vi "requestStop.vi"(8 "error in (no error)":errorcluster, 11 "MsgUserEventStopMechanism In":refnum<class "MsgUETaskChannel.lvclass">) -> (0 "error out":errorcluster, 3 "MsgUserEventStopMechanism Out":refnum<class "MsgUETaskChannel.lvclass">)   [LabVIEW 2023, in "TLC_Daemon.lvlib" / "MsgUETaskChannel.lvclass"]
doc: "Triggers a stop request for a target task."
uses:
  MsgUETaskChannel.lvclass
  MsgUETaskChannel.lvclass/MsgUETaskChannel.ctl
  Ctrls/msg.ctl
  TLC_Daemon.lvlib
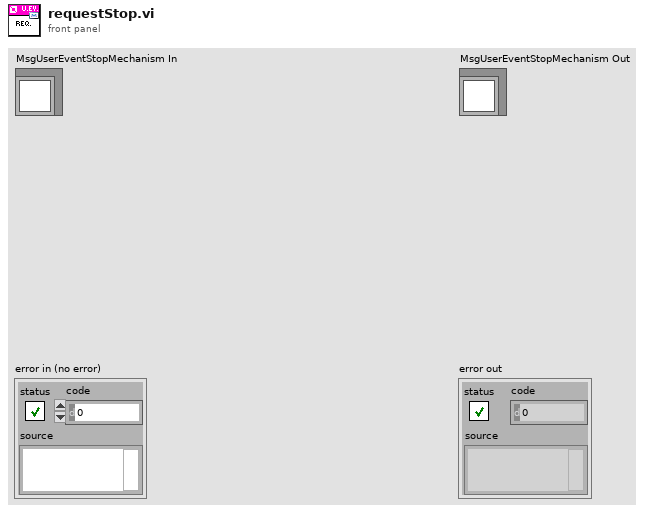
[diagram p1: front panel]
types:
  T1 = typedef "TLC_Daemon.lvlib/msg.ctl" = cluster{"message":string, "data":variant}
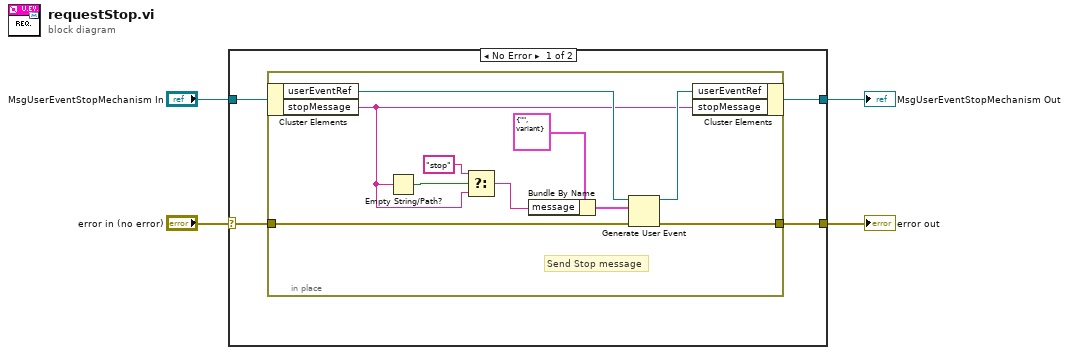
[diagram p0: block diagram]
diagram:
  n1 = case shown="No Error" "error in (no error)" {
    selector: "error in (no error)" -> [w7 w20]
    tunnel: [w6 w20] -> w3
    tunnel: "MsgUserEventStopMechanism In" -> [w8 w19]
    tunnel: [w5 w19] -> w1
    frame No Error {
      n2 = in-place {
        in-place-border: w7 -> [w16]
        in-place-border: [w15] -> w6
        # "Send Stop message"
        n3 = in-place-cluster #1(w8) -> ("userEventRef"=w18:refnum<user-event>, "stopMessage"=w11:string)
        n4 = Empty String/Path?(string/path=w11) -> (empty?=w12:bool)
        n5 = Select(t="stop", s=w12, f=w11) -> (s? t:f=w10:string)
        n6 = Bundle By Name(cluster=T1 {"message"="", "data"=variant} ("msg"), "message"=w10) -> (w14:T1)
        n7 = Generate User Event(user event=w18, event data cluster=w14, error in=w16) -> (user event out=w17:refnum<user-event>, error out=w15:errorcluster)  [unwired: 1 in]
        n8 = in-place-cluster #1("userEventRef"=w17, "stopMessage"=w11) -> (w5:refnum<class "MsgUETaskChannel.lvclass">)
      }
    }
    frame Error {
    }
  }
  "error out" <- w3
  "MsgUserEventStopMechanism Out" <- w1
